vi "Generate Check Event.vi"(8 "error in (no error)":errorcluster) -> (0 "error out":errorcluster)   [LabVIEW 2017, in "WebServiceImporter.lvlib" / "Main Panel.lvlib" / "Select Methods.lvlib" / "Events.lvlib"]
uses:
  <vilib>/Platform/WebService/Main Panel/Pages/Select Methods/Events/Events.lvlib
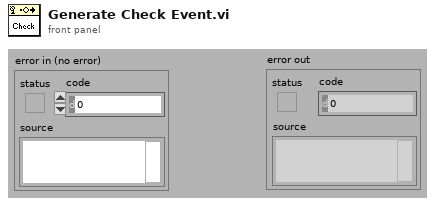
[diagram p1: front panel]
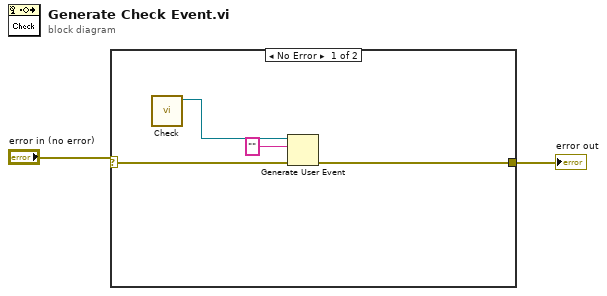
[diagram p0: block diagram]
diagram:
  n1 = case shown="No Error" "error in (no error)" {
    selector: "error in (no error)" -> [w6 w7]
    tunnel: [w4 w7] -> w1
    frame No Error {
      n2 = call <vilib>:"Check.vi"() -> ("user event (out)"=w3:refnum<user-event>)  [unwired: 10 in, 1 out]
      n3 = Generate User Event(user event=w3, event data cluster="" ("event data"), error in=w6) -> (error out=w4:errorcluster)  [unwired: 1 in, 1 out]
    }
    frame Error {
    }
  }
  "error out" <- w1
